vi "Brute Force Dark Current Primary Logic Body.vi"(0 "Barcodes in":string[](array[string]), 1 "stop":bool, 2 "First Tube #":i32, 5 "VISA Refnum in":refnum<visa-resource-name>, 6 "Number of Tubes":i32, 7 "Channel #":i32) -> (10 "Actual Voltage Level (V)":dbl format="%#_13g", 11 "Individual Tube Current (Nano Amps)":dbl[](array[numeric]), 12 "Actual Current Limit (nA)":dbl format="%#_13g", 13 "Mesurnment  Iteration":i32, 14 "Power Supply Trip":bool, 19 "Failed Tubes":string[](array[string]))   [LabVIEW 2020]
uses:
  Program Files/National Instruments/LabVIEW 2018/instr.lib/CAEN PSM/CAEN PSM.lvlib
panel:
  out "error out":errorcluster
  out "BoardHandle out":T1
  # "Pin in"
  # "Pin out"
  # "No pin"
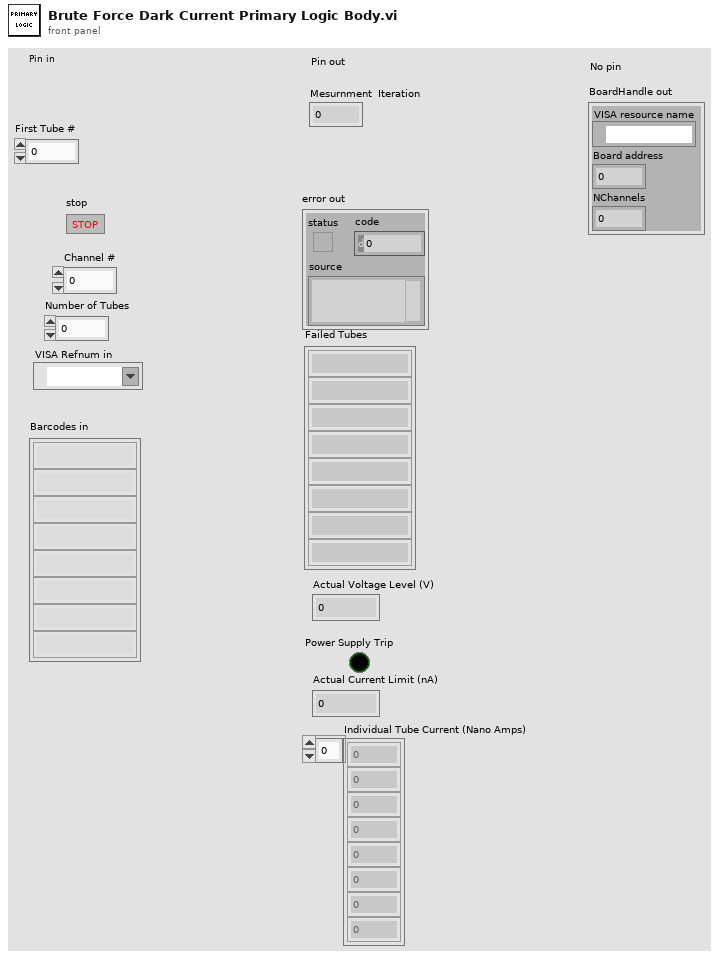
[diagram p1: front panel]
types:
  T1 = cluster{"VISA resource name":refnum<visa-resource-name>, "Board address":u8, "NChannels":u8}
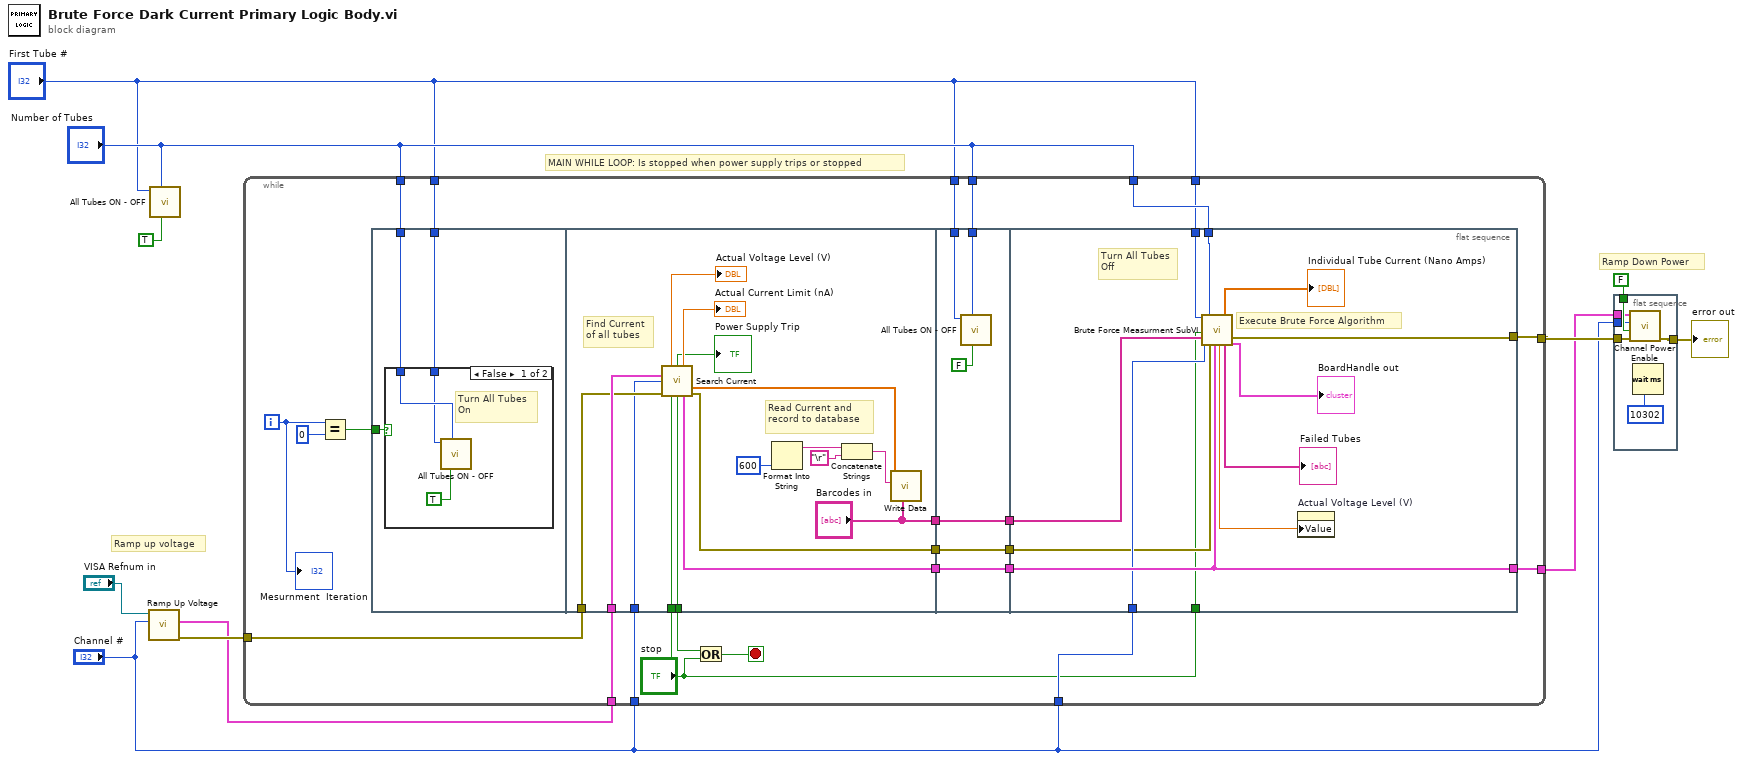
[diagram p0: block diagram]
diagram:
  # "Ramp Down Power"
  # "MAIN WHILE LOOP: Is stopped when power supply trips or stopped"
  # "Ramp up voltage"
  n1 = call "Ramp Up Voltage.vi"("Channel # in"="Channel #", "VISA Refnum in"="VISA Refnum in") -> ("error out"=w8:errorcluster, "BoardHandle out"=w7:T1)  [unwired: 8 in]
  n2 = call "All Tubes ON - OFF.vi"("Tubes ON/OFF"=TRUE ("Activate: 1\nDeactivate: 0"), "Number of tubes"="Number of Tubes", "First Tube"="First Tube #") -> ()  [unwired: 9 in]
  n3 = while {
    tunnel: "Number of Tubes" -> [w35]
    tunnel: "Number of Tubes" -> [w16]
    tunnel: "Channel #" -> [w34]
    tunnel: w7 -> [w33]
    tunnel: "Number of Tubes" -> [w32]
    tunnel: w8 -> [w31]
    tunnel: [w28] -> w9
    tunnel: [w27] -> w11
    tunnel: "Channel #" -> [w26]
    tunnel: "First Tube #" -> [w14]
    tunnel: "First Tube #" -> [w13]
    tunnel: "First Tube #" -> [w12]
    i -> [w25]
    stop <- w29 stop-if-true
    n4 = Equal?(x=w25, y=0) -> (x = y?=w23:bool)
    n5 = flat-sequence {
      tunnel: w32 -> [w38]
      tunnel: w23 -> [w37]
      tunnel: w14 -> [w36]
      tunnel: w34 -> [w45]
      tunnel: w33 -> [w48]
      tunnel: [w52] -> w18
      tunnel: [w50] -> w20
      tunnel: ["Barcodes in"] -> w22
      tunnel: w31 -> [w47]
      tunnel: [w44] -> w30
      tunnel: "stop" -> [w42]
      tunnel: w22 -> [w62]
      tunnel: [w62] -> w21
      tunnel: w20 -> [w61]
      tunnel: [w61] -> w19
      tunnel: w18 -> [w60]
      tunnel: [w60] -> w17
      tunnel: w16 -> [w58]
      tunnel: w13 -> [w57]
      tunnel: w35 -> [w73]
      tunnel: w21 -> [w74]
      tunnel: w19 -> [w72]
      tunnel: w17 -> [w66]
      tunnel: [w72] -> w28
      tunnel: [w65] -> w27
      tunnel: w26 -> [w67]
      tunnel: "stop" -> [w64]
      tunnel: w12 -> [w63]
      frame #0 {
        n6 = case shown="False" w37 {
          tunnel: w38 -> [w41 _]
          tunnel: w36 -> [w39 _]
          frame False {
            # "Turn All Tubes \nOn"
            n7 = call "All Tubes ON - OFF.vi"("Tubes ON/OFF"=TRUE, "Number of tubes"=w41, "First Tube"=w39) -> ()  [unwired: 9 in]
          }
          frame True {
          }
        }
      }
      frame #1 {
        # "Find Current\nof all tubes"
        # "Read Current and  record to database"
        n8 = call "Search Current.vi"("BoardHandle in"=w48, "Channel # in"=w45, "error in (no error)"=w47, "Stop Program Search Current"=w42) -> ("Actual Voltage Level (V)"=→"Actual Voltage Level (V)":dbl, "Power Supply Trip"=w44:bool, "Actual Current Limit (nA)"=→"Actual Current Limit (nA)":dbl, "Array"=w51:dbl[], "BoardHandle out 2"=w50:T1, "error out"=w52:errorcluster)  [unwired: 6 in]
        "Power Supply Trip" <- w44
        n9 = Format Into String(600 ("input 1")) -> (resulting string=w55:string)  [unwired: 3 in, 1 out]
        n10 = Concatenate Strings(w55, "\r") -> (w56:string)
        n11 = call "Write Data.vi"("Barcodes"="Barcodes in", "Array"=w51, "String"=w56) -> ()  [unwired: 9 in]
      }
      frame #2 {
        n12 = call "All Tubes ON - OFF.vi"("Tubes ON/OFF"=FALSE ("Activate: 1\nDeactivate: 0"), "Number of tubes"=w58, "First Tube"=w57) -> ()  [unwired: 9 in]
      }
      frame #3 {
        # "Execute Brute Force Algorithm"
        # "Turn All Tubes\nOff"
        n13 = call "Brute Force Measurment SubVI.vi"("First Tube #"=w63, "Stop Program Brute Force"=w64, "Barcodes in"=w74, "Channel # in"=w67, "Last Tube #"=w73, "error in (no error)"=w66, "BoardHandle in"=w72) -> ("Actual Voltage Level (V) 2"=w71:dbl, "Individual Tube Current (Nano Amps)"=→"Individual Tube Current (Nano Amps)":dbl[], "Failed Tubes"=→"Failed Tubes":string[], "error out"=w65:errorcluster, "BoardHandle out"=→"BoardHandle out":T1)  [unwired: 8 in]
        n14 = property on="Actual Voltage Level (V)" class="DigNum (strict)"("Value"=w71) -> ()  [unwired: 2 in, 2 out]
      }
    }
    n15 = Or(x=w30, y="stop") -> (x .or. y?=w29:bool)
    "Mesurnment  Iteration" <- w25
  }
  n16 = flat-sequence {
    tunnel: w11 -> [w80]
    tunnel: FALSE ("Enable (OFF)") -> [w79]
    tunnel: w9 -> [w78]
    tunnel: "Channel #" -> [w77]
    tunnel: [w76] -> w4
    frame #0 {
      n17 = call "Channel Power Enable.vi"("error in (no error)"=w80, "Enable (OFF)"=w79, "Channel (0)"=w77, "BoardHandle"=w78) -> ("error out"=w76:errorcluster)  [unwired: 6 in, 1 out]
      n18 = Wait (ms)(milliseconds to wait=u32 10302) -> ()  [unwired: 1 out]
    }
  }
  "error out" <- w4
